vi "FGV_Open binary video refs.vi"(8 "error in (no error)":errorcluster, 10 "Function":T1, 11 "Filtered Array in":path[](array[path])) -> (0 "error out":errorcluster, 3 "Cam Binary Videos (ref)":refnum<file>[](array[refnum]))   [LabVIEW 2013]
uses:
  Functional Imaging Viewer/Typedefs/Get-Set-Clear Control.ctl
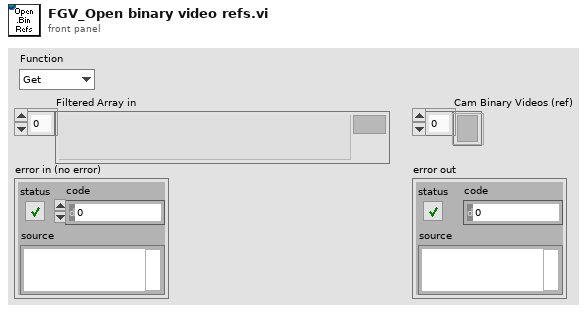
[diagram p1: front panel]
types:
  T1 = typedef "Get-Set-Clear Control.ctl" = enum16{"Get", "Set", "Clear"}
  T2 = enum16{"open", "replace", "create", "open or create", "replace or create", "replace or create with confirmation"}
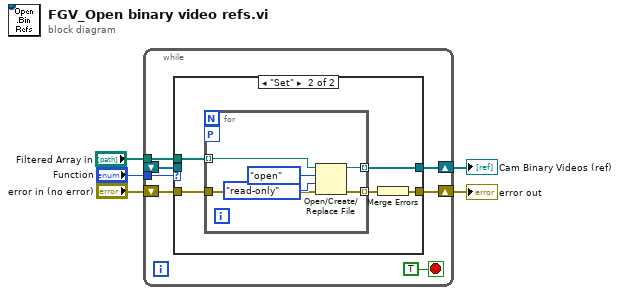
[diagram p0: block diagram]
diagram:
  n1 = while {
    tunnel: "Filtered Array in" -> [w10]
    tunnel: "Function" -> [w8]
    shift-right: [w11] -> w4
    shift-left: _ -> [w7]
    shift-right: [w12] -> w5
    shift-left: "error in (no error)" -> [w6]
    stop <- TRUE stop-if-true
    n2 = case shown="\"Set\"" w8 {
      tunnel: [w13 w19] -> w12
      tunnel: w6 -> [w13 w17]
      tunnel: [w14 w16] -> w11
      tunnel: w10 -> [_ w15]
      tunnel: w7 -> [w14 _]
      frame "Get", Default {
      }
      frame "Set" {
        n3 = for {
          tunnel: w15 -> [w23] mode=indexing
          tunnel: [w22] -> w16 mode=indexing
          tunnel: w17 -> [w21]
          tunnel: [w20] -> w18 mode=indexing
          workers-P: _ -> [_]
          n4 = Open/Create/Replace File(file path (use dialog)=w23, error in=w21, operation (0:open)=T2."open", access (0:read/write)=enum16{"read/write", "read-only", "write-only"}."read-only") -> (refnum out=w22:refnum<file>, error out=w20:errorcluster)  [unwired: 2 in, 1 out]
        }
        n5 = Merge Errors(w18) -> (w19:errorcluster)
      }
    }
  }
  "Cam Binary Videos (ref)" <- w4
  "error out" <- w5
